vi "Creators Self Queue Alias.vi"(11 "Event jettl in":refnum<class "Event jettl.lvclass">) -> (2 "Self Queue Alias":string, 3 "Event jettl out":refnum<class "Event jettl.lvclass">)   [LabVIEW 2021, in "jettl.lvlib" / "Event jettl.lvclass"]
uses:
  Event jettl.lvclass
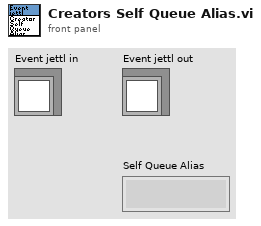
[diagram p1: front panel]
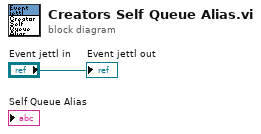
[diagram p0: block diagram]
diagram:
  "Event jettl out" <- "Event jettl in"
